vi "LEBITVacuum.GetEnable.vi"(1 "EnableValuePLC":string, 5 "quality in":i32) -> (19 "quality out":i32)   [LabVIEW 2014, in "LEBITVacuum.lvlib"]
uses:
  LEBITVacuum.lvlib
  CS_Core/CSSystem/CoreDefs/CoreDefs.call_type.ctl
  CS_Core/BaseProcess/BaseProcess.descriptor string definition.ctl
  CS_Core/CSSystem/CoreDefs/CoreDefs.rawDataType.ctl
  CSlibraries/UtilityLib/UtilityLib.valueStatus.ctl
  CS_Core/CSSystem/CoreLib/CoreLib.string 2 byte array.vi
  CS_Core/CSSystem/CoreLib/CoreLib.byte array 2 short.vi
  CS_Core/CSSystem/CoreLib/CoreLib.lvlib
  CSlibraries/UtilityLib/UtilityLib.lvlib
  CS_Core/BaseProcess/BaseProcess.lvlib
panel:
  in  "call cluster in":T1={"Object"="", "Selector"="", "CallType"=enum."synchronous", "Async Object"="", "Async Selector"="", "Data Descriptor"="", "Data"=[], "Error #"=0, "Expire"=0}
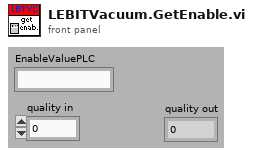
[diagram p1: front panel]
types:
  T1 = typedef "CoreDefs.call_type.ctl" = cluster{"Object":string, "Selector":string, "CallType":enum16{"simple", "synchronous", "asynchronous"}, "Async Object":string, "Async Selector":string, "Data Descriptor":T2, "Data":T3, "Error #":i32, "Expire":u32}
  T2 = typedef "BaseProcess.lvlib/BaseProcess.descriptor string definition.ctl" = string
  T3 = typedef "CoreDefs.rawDataType.ctl" = i8[]
  T4 = typedef "UtilityLib.lvlib/UtilityLib.valueStatus.ctl" = enum16{"no info available", "stand by/off", "on", "warning", "alarm/malfunction", "not implemented", "user action required", "important information", "system default", "control default", "indicator default", "button default"}
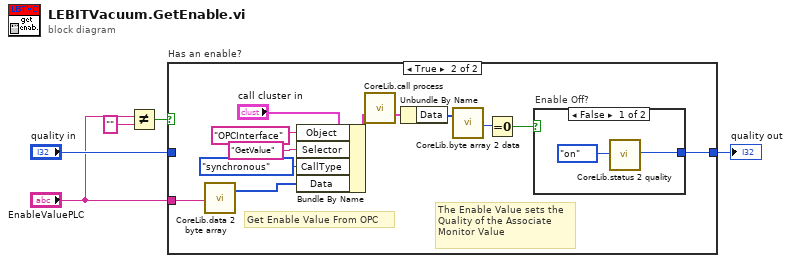
[diagram p0: block diagram]
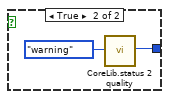
[diagram p3: hidden frame]
diagram:
  n1 = Not Equal?(x="EnableValuePLC", y="") -> (x != y?=w1:bool)
  n2 = case "Has an enable?" shown="True" w1 {
    tunnel: [w6 w17] -> w4
    tunnel: "quality in" -> [w6 _]
    tunnel: "EnableValuePLC" -> [_ w18]
    frame False {
    }
    frame True {
      # "The Enable Value sets the \nQuality of the Associate\nMonitor Value"
      # "Get Enable Value From OPC"
      n3 = call-poly "CoreLib.data 2 byte array.vi"("string"=w18) -> ("byteArray out"=w13:T3)  [unwired: 18 in]
      n4 = Bundle By Name(cluster="call cluster in", "Object"="OPCInterface", "Selector"="GetValue" ("string"), "CallType"=enum16{"simple", "synchronous", "asynchronous"}."synchronous", "Data"=w13) -> (w16:T1)
      n5 = call "CoreLib.call process.vi"("call cluster in"=w16) -> ("call cluster out"=w10:T1)  [unwired: 13 in, 1 out]
      n6 = Unbundle By Name(w10) -> ("Data"=w9:T3)
      n7 = call-poly "CoreLib.byte array 2 data.vi"("byteArray"=w9) -> ("i16"=w7:i16)  [unwired: 16 in, 2 out]
      n8 = Equal To 0?(x=w7) -> (x = 0?=w8:bool)
      n9 = case "Enable Off?" shown="False" w8 {
        tunnel: [w19 w21] -> w17
        frame False {
          n10 = call "CoreLib.status 2 quality.vi"("valueStatus"=UtilityLib.valueStatus."on") -> ("quality"=w19:i32)  [unwired: 18 in]
        }
        frame True {
          n11 = call "CoreLib.status 2 quality.vi"("valueStatus"=UtilityLib.valueStatus."warning") -> ("quality"=w21:i32)  [unwired: 18 in]
        }
      }
    }
  }
  "quality out" <- w4
